vi "Alarma parpadeante (elemento).vi"(7 "Color ON2":u32(colorbox), 8 "Color ON1":u32(colorbox), 9 "Color OFF":u32(colorbox), 10 "Cambio de color":dbl, 11 "Buffer de error":dbl) -> (3 "Color (alarma)":u32(colorbox))   [LabVIEW 2013]
panel:
  in  "Tiempo acumulado":u32
  in  "Tiempo actual":u32
  in  "Tiempo anterior":u32
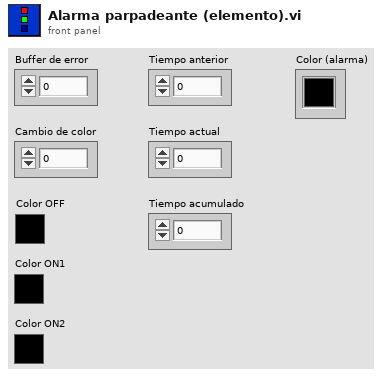
[diagram p1: front panel]
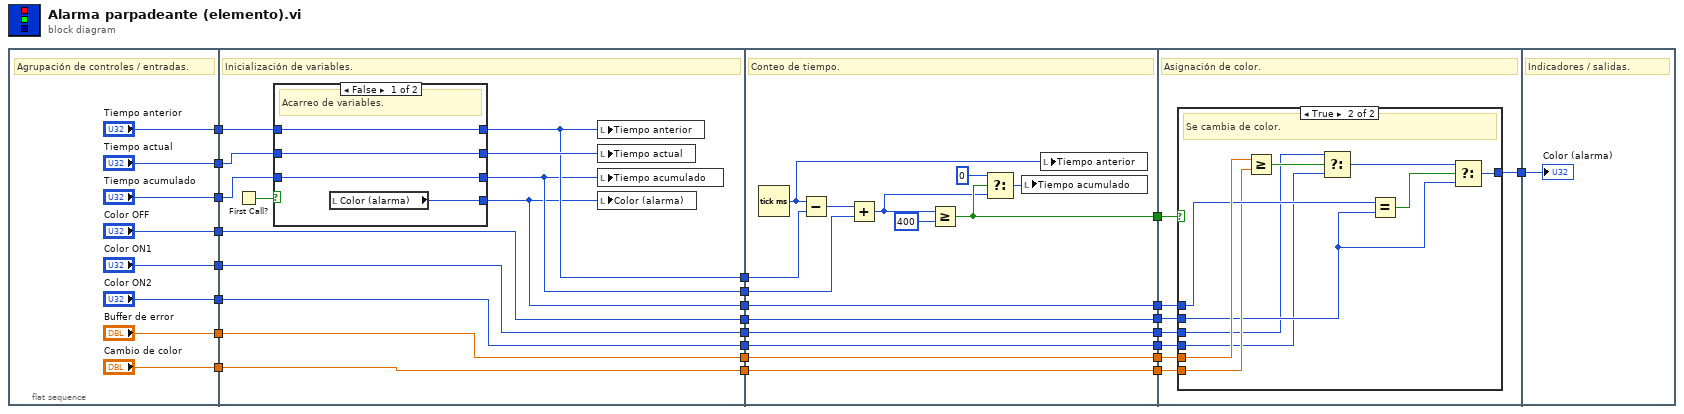
[diagram p0: block diagram]
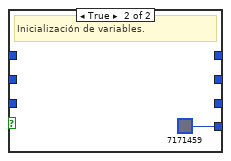
[diagram p2: hidden frame]
diagram:
  n1 = flat-sequence {
    tunnel: ["Buffer de error"] -> w21
    tunnel: ["Tiempo anterior"] -> w16
    tunnel: ["Tiempo actual"] -> w15
    tunnel: ["Tiempo acumulado"] -> w14
    tunnel: ["Cambio de color"] -> w12
    tunnel: ["Color OFF"] -> w9
    tunnel: ["Color ON1"] -> w8
    tunnel: ["Color ON2"] -> w7
    tunnel: [w43] -> w24
    tunnel: [w42] -> w23
    tunnel: w21 -> [w41]
    tunnel: [w41] -> w20
    tunnel: [w40] -> w18
    tunnel: w16 -> [w39]
    tunnel: w15 -> [w37]
    tunnel: w14 -> [w38]
    tunnel: w12 -> [w36]
    tunnel: [w36] -> w11
    tunnel: w9 -> [w33]
    tunnel: w8 -> [w35]
    tunnel: w7 -> [w34]
    tunnel: [w35] -> w6
    tunnel: [w34] -> w5
    tunnel: [w33] -> w1
    tunnel: w24 -> [w65]
    tunnel: w23 -> [w63]
    tunnel: [w60] -> w22
    tunnel: w20 -> [w61]
    tunnel: [w61] -> w19
    tunnel: w18 -> [w56]
    tunnel: [w56] -> w17
    tunnel: w11 -> [w54]
    tunnel: [w54] -> w10
    tunnel: w6 -> [w53]
    tunnel: w5 -> [w52]
    tunnel: [w53] -> w4
    tunnel: [w52] -> w3
    tunnel: [w51] -> w2
    tunnel: w1 -> [w51]
    tunnel: w22 -> [w72]
    tunnel: w19 -> [w73]
    tunnel: w17 -> [w71]
    tunnel: [w70] -> w13
    tunnel: w10 -> [w69]
    tunnel: w4 -> [w68]
    tunnel: w3 -> [w67]
    tunnel: w2 -> [w66]
    tunnel: w13 -> [w85]
    frame #0 {
      # "Agrupación de controles / entradas."
    }
    frame #1 {
      # "Inicialización de variables."
      n2 = First Call?() -> (First Call?: T/F=w45:bool)
      n3 = case shown="False" w45 {
        tunnel: [w49 u32 7171459] -> w40
        tunnel: [w48 _] -> w43
        tunnel: [w47 _] -> w44
        tunnel: [w46 _] -> w42
        tunnel: w39 -> [w48 _]
        tunnel: w37 -> [w47 _]
        tunnel: w38 -> [w46 _]
        frame False {
          # "Acarreo de variables."
          n4 = local read "Color (alarma)"() -> (w49:u32)
        }
        frame True {
          # "Inicialización de variables."
        }
      }
      n5 = local write "Tiempo anterior"(w43) -> ()
      n6 = local write "Tiempo actual"(w44) -> ()
      n7 = local write "Tiempo acumulado"(w42) -> ()
      n8 = local write "Color (alarma)"(w40) -> ()
    }
    frame #2 {
      # "Conteo de tiempo."
      n9 = Tick Count (ms)() -> (millisecond timer value=w55:u32)
      n10 = Subtract(x=w55, y=w65) -> (x-y=w64:u32)
      n11 = Add(x=w64, y=w63) -> (x+y=w58:u32)
      n12 = Greater Or Equal?(x=w58, y=u32 400) -> (x >= y?=w60:bool)
      n13 = Select(t=u32 0, s=w60, f=w58) -> (s? t:f=w57:u32)
      n14 = local write "Tiempo acumulado"(w57) -> ()
      n15 = local write "Tiempo anterior"(w55) -> ()
    }
    frame #3 {
      # "Asignación de color."
      n16 = case shown="True" w72 {
        tunnel: w73 -> [_ w81]
        tunnel: w71 -> [w74 w80]
        tunnel: [w74 w79] -> w70
        tunnel: w69 -> [_ w78]
        tunnel: w68 -> [_ w76]
        tunnel: w67 -> [_ w75]
        tunnel: w66 -> [_ w77]
        frame False {
          # "Se acarrea el dato."
        }
        frame True {
          # "Se cambia de color."
          n17 = Greater Or Equal?(x=w81, y=w78) -> (x >= y?=w84:bool)
          n18 = Select(t=w76, s=w84, f=w75) -> (s? t:f=w83:u32)
          n19 = Equal?(x=w80, y=w77) -> (x = y?=w82:bool)
          n20 = Select(t=w83, s=w82, f=w77) -> (s? t:f=w79:u32)
        }
      }
    }
    frame #4 {
      # "Indicadores / salidas."
      "Color (alarma)" <- w85
    }
  }
